vi "1.3.4-Paths.vi"(11 "allowed proximity squared":i16=400) -> ()   [LabVIEW 2010]
uses:
  <vilib>/rvi/DataTransferAndStorage/Container/XNode/niFpgaContainer.xnode
  Unsorted Files from Athena/athena FPGA globals.vi
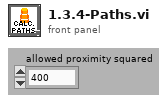
[diagram p1: front panel]
types:
  T1 = enum16{"confirm check sum", "check status byte", "read measured values", "confirm measurement", "confirm command", "read message length", "read address", "wait for \"02\""}
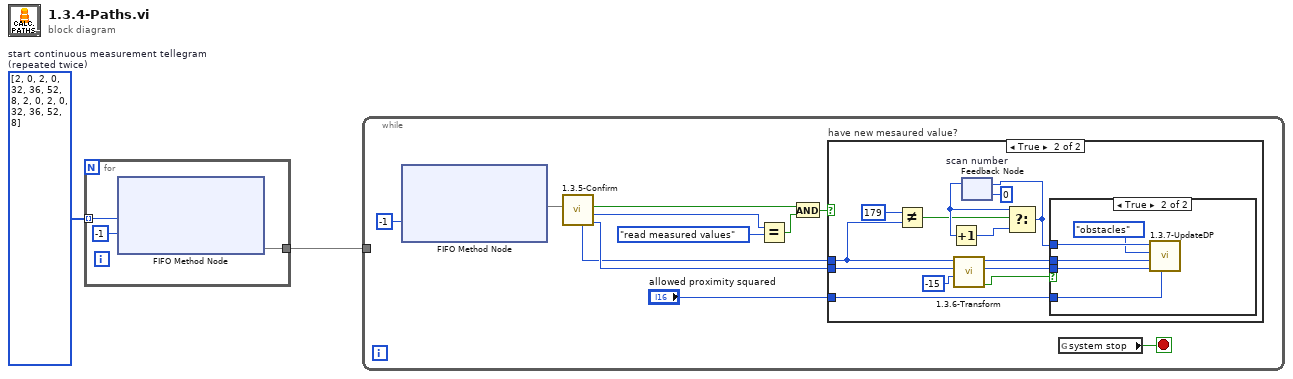
[diagram p0: block diagram]
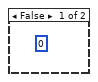
[diagram p2: hidden frame]
diagram:
  w1 = u8[] [2, 0, 2, 0, 32, 36, 52, 8, 2, 0, 2, 0, 32, 36, 52, 8]  # start continuous measurement tellegram (repeated twice)
  n1 = for {
    tunnel: w1 -> [w5] mode=indexing
    tunnel: [w3] -> w2
    n2 = xnode ("FIFO Method Node")("Element"=w5, "Timeout"=-1) -> ("Timed Out?"=w3)  [unwired: 1 in, 1 out]
  }
  n3 = while {
    tunnel: w2 -> [_]
    stop <- w7 stop-if-true
    n4 = xnode ("FIFO Method Node")("Timeout"=-1) -> ("Element"=w16)  [unwired: 1 in, 2 out]
    n5 = call "1.3.5-Confirm.vi"("LIDAR raw data"=w16) -> ("last measured value"=w15:u16, "parser state"=w14:T1, "new value?"=w13:bool, "angle"=w9:u8)  [unwired: 7 in]
    n6 = Equal?(x=w14, y=T1."read measured values" ("parser state")) -> (x = y?=w10:bool)
    n7 = And(x=w13, y=w10) -> (x .and. y?=w12:bool)
    n8 = case "have new mesaured value?" shown="True" w12 {
      tunnel: w15 -> [_ w29]
      tunnel: w9 -> [_ w22]
      tunnel: "allowed proximity squared" -> [_ w17]
      frame False {
        (unwired) u8 0 ("y")
      }
      frame True {
        n9 = Not Equal?(x=u8 179, y=w22) -> (x != y?=w23:bool)
        n10 = call "1.3.6-Transform.vi"("Lidar Vertical Position"=i8 -15, "Lidar Distance"=w29, "Lidar Scan Angle"=w22) -> ("Is object?"=w26:bool, "Robot Y"=w27:i16, "Lidar X = Robot X"=w28:i16)  [unwired: 3 in, 3 out]
        n11 = feedback #1 "scan number"(u8 0 ("y")) -> (w25:u8)
        n12 = Increment(x=w25) -> (x+1=w24:u8)
        n13 = Select(t=w25, s=w23, f=w24) -> (s? t:f=w20:u8)
        n14 = feedback-in #1(w20) -> ()
        n15 = case shown="True" w26 {
          tunnel: w28 -> [_ w34]
          tunnel: w27 -> [_ w33]
          tunnel: w20 -> [_ w32]
          tunnel: w17 -> [_ w30]
          frame False {
          }
          frame True {
            n16 = call "1.3.7-UpdateDP.vi"("allowed proximity squared"=w30, "Robot Y"=w33, "Robot X"=w34, "update lines or objects"=enum16{"lines", "obstacles"}."obstacles", "Scan Number"=w32) -> ()  [unwired: 7 in]
          }
        }
      }
    }
    n17 = global read "athena FPGA globals.vi" "system stop"() -> (w7:bool)
  }
